vi "LVClass_HasoSlopes ctor from ModalCoef.vi"(0 "HasoSlopes (const)":refnum<class "HasoSlopes.lvclass">, 5 "ModalCoef":refnum<class "ModalCoef.lvclass">, 7 "Haso configuration file":path, 11 "error in (no error)":errorcluster) -> (4 "HasoSlopes (new)":refnum<class "HasoSlopes.lvclass">, 6 "ModalCoef (dup)":refnum<class "ModalCoef.lvclass">, 15 "error out":errorcluster)   [LabVIEW 2020, in "HasoSlopes.lvclass"]
doc: "HasoSlopes constructor from ModalCoef.\n\n<B>HasoSlopesIn</B> : Constant Pointer to HasoSlopes object.\n<B>HasoSlopesOut</B> : Constant Pointer to HasoSlopes object.\n<B>ModalCoef</B> : ModalCoef object.\n<B>config_file_path</B> : Absolute path to Haso configuration file."
uses:
  HasoSlopes.lvclass
  ModalCoef/ModalCoef.lvclass
  Controls/Handle creation.ctl
  HasoSlopes.lvclass/HasoSlopes.ctl
  ModalCoef/LVClass_ModalCoef Read ModalCoef.vi
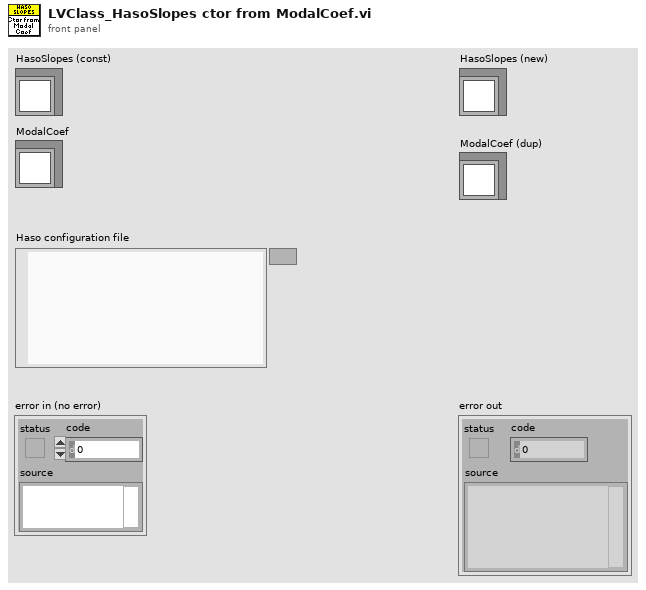
[diagram p1: front panel]
types:
  T1 = typedef "Handle creation.ctl" = enum16{"By ctor", "By write function"}
  T2 = typedef "ClassID.ctl" = i64
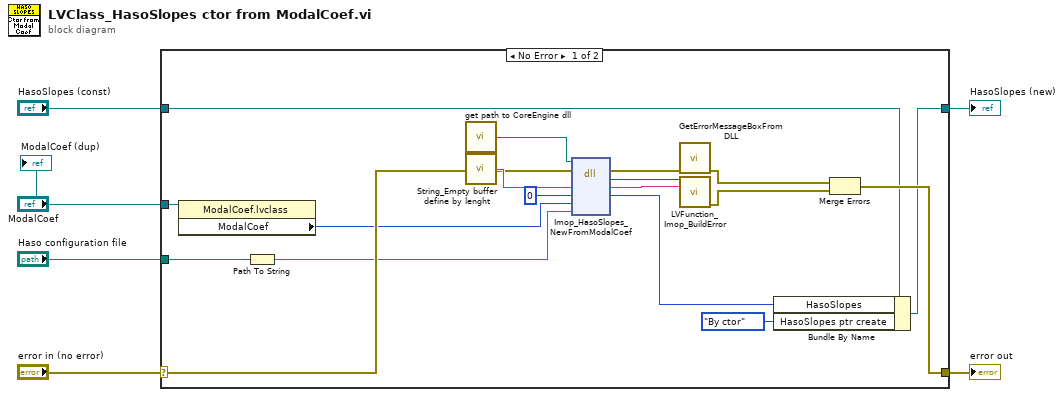
[diagram p0: block diagram]
diagram:
  n1 = case shown="No Error" "error in (no error)" {
    selector: "error in (no error)" -> [w17 w26]
    tunnel: [w16 w26] -> w5
    tunnel: [w14 w25] -> w3
    tunnel: "HasoSlopes (const)" -> [w15 w25]
    tunnel: "ModalCoef" -> [w11 _]
    tunnel: "Haso configuration file" -> [w10 _]
    frame No Error {
      n2 = property class="ModalCoef.lvclass"(reference=w11) -> ("ModalCoef"=w7:T2)  [unwired: 1 in, 2 out]
      n3 = Path To String(path=w10) -> (string=w9:string)
      n4 = call "get path to CoreEngine dll.vi"() -> ("path to wavekit library"=w20:path)  [unwired: 14 in, 1 out]
      n5 = call "String_Empty buffer define by lenght.vi"() -> ("Empty buffer"=w21:string)  [unwired: 1 in]
      n6 = dll-call lib="D:/FLE/0.Code/CoreEngine4_Suite/LV2011_interface/DLLs/c_interface_vc100.dll" fn="Imop_HasoSlopes_NewFromModalCoef"(path in=w20, error in=w17, "Message"=w21, "HasoSlopes"=0, "Modal Coef"=w7, "HASO configuration path"=w9) -> (error out=w24:errorcluster, "return type"=w22:i32, "Message"=w23:string, "HasoSlopes"=w8:i64)  [unwired: 3 in, 1 out]
      n7 = call "GetErrorMessageBoxFromDLL.vi"("error IN"=w24) -> ("error OUT"=w19:errorcluster)  [unwired: 10 in]
      n8 = call "LVFunction_Imop_BuildError.vi"("code"=w22, "String to Prepend to source (\"\")"=w23) -> ("error out"=w18:errorcluster)  [unwired: 13 in]
      n9 = Bundle By Name(cluster=w15, "HasoSlopes"=w8, "HasoSlopes ptr create"=Handle_creation."By ctor") -> (w14:refnum<class "HasoSlopes.lvclass">)
      n10 = Merge Errors(w19, w18) -> (w16:errorcluster)
    }
    frame Error {
    }
  }
  "error out" <- w5
  "HasoSlopes (new)" <- w3
  "ModalCoef (dup)" <- "ModalCoef"
